vi "Dashboard Main.vi"() -> ()   [LabVIEW 2015]
uses:
  <vilib>/Utility/miscctls.llb/LVRowAndColumnTypeDef.ctl
  <vilib>/event_ctls.llb/eventvkey.ctl
  <vilib>/Rock Robotics/Network Tables/NT Read Boolean.vi
  <vilib>/Rock Robotics/WPI/Dashboard/WPI_DashboardLogging Global.vi
  <vilib>/Rock Robotics/Network Tables/NT Read Numeric Array.vi
  <vilib>/Utility/config.llb/Write Key (String).vi
  <vilib>/Utility/config.llb/Write Key (I32).vi
  <vilib>/Rock Robotics/Network Tables/NT Write Boolean.vi
  <vilib>/Utility/config.llb/NI_LVConfig.lvlib
panel:
  out "Gyro":dbl(knob)=-1.8413610199999755 scale=-180.0..180.0
  in  "Auto Delay (s)":dbl
  in  "Select Auto":string(combo)="Cross" caption="I don't care if I have the routine you want,\nCLICK ME AGAIN"
  out "Binary Image":T1(plugin-control)
  in  "TCP":refnum<k5>
  out "Camera IP":string="0.0.0.0"
  out "Image Message":string="Timeout in Camera Communications"
  in  "Dashboard Tab":T2(tab)
  in  "Cross Back":bool
  in  "Defense":u16(ring) items=["Default", "Low Bar", "Portcullis", "Cheval de Frise", "Ramparts", "Moat", "Drawbridge", "Sally Port", "Rock Wall", "Rough Terrain"]
  in  "Joystick Drive":u16(ring) items=["TANK DRIVE", "LEFT ARCADE", "RIGHT ARCADE"]
  in  "Auto Routine":u16(ring)=1 items=["Do Nothing", "Cross", "Spybot", "Reach", "Test"]
  in  "Shoot?":bool=TRUE
  in  "Defense Position":dbl=1.0 min=0.0 max=5.0 format="%#_1g"
  in  "Camera Settings":T3={"Frame Rate"=15, "Compression"=30, "Size"=1} {"Frame Rate" scale=1.0..30.0; "Size" items=["640x480", "320x240", "160x120"]}
  out "Mode":T4(ring)=enum."Disconnected"
  in  "DB Camera Config":bool
  out "fps":dbl=0.2739425816348893 format="%#.1g"
  out "Mbps":dbl=2.2448263767099263e-06 format="%#.1g"
  out "Mbps LED":bool
  in  "Rec Mode":enum32{"Stop", "Record", "Playback"}(radio)
  out "NT Connection":bool=TRUE
  in  "Vision":u16(ring)=2 items=["Camera Off", "USB Camera SW", "USB Camera HW", "IP Camera"]
  out "Time Left":string="135"
  out "Background":bool=TRUE
  in  "DB/String 9":string
  in  "DB/String 8":string
  in  "DB/String 7":string
  in  "DB/String 6":string
  in  "DB/String 5":string
  in  "DB/String 4":string
  in  "DB/String 3":string
  in  "DB/String 2":string
  in  "DB/String 1":string
  in  "DB/String 0":string
  in  "DB/Slider 0":dbl(slide)=1.0 caption="Intake Roller Speed" min=0.0 max=1.0 scale=0.0..1.0
  in  "DB/Slider 1":dbl(slide) scale=0.0..5.0
  in  "DB/Slider 2":dbl(slide) scale=0.0..5.0
  in  "DB/Slider 3":dbl(slide) scale=0.0..5.0
  out "DB/LED 3":bool
  out "DB/LED 2":bool
  out "DB/LED 1":bool
  out "DB/LED 0":bool
  in  "DB/Button 3":bool
  in  "DB/Button 2":bool
  in  "DB/Button 1":bool
  in  "DB/Button 0":bool caption="New Name"
  in  "Test Slider":dbl(slide) scale=0.0..100.0 scale format="%#_3g"
  in  "On/Off":bool caption="Solenoid"
  in  "Test Name":u16(ring) items=["Select the test to run..."]
  in  "Test Tree":string(tree)
  in  "Motor":cluster{"Value":dbl, "Enable":bool} {"Value" scale=-1.0..1.0 scale format="%#_3g"}
  out "Progress":T5 {"Test Progress" scale=0.0..100.0}
  in  "Rev/Fwd":cluster{"Forward":bool, "Reverse":bool}
  in  "Test Ring":u16(ring) items=["Monochrome", "Color"]
  out "Cmd Status":string
  in  "Execute Command":bool
  in  "Command Params":string[][](table)
  in  "Command Selection":i32(listbox)
  in  "CheckList":i32(listbox)
  out "Tree":string(tree)
  out "Camera Image":T1(plugin-control)
  # "1 Low Bar\n2 Porticullis\n3 Cheval De Frise\n4 Ramparts\n5 Moat\n6 Drawbridge\n7 Sally Port\n8 Rock Wall\n9 Rough Terain"
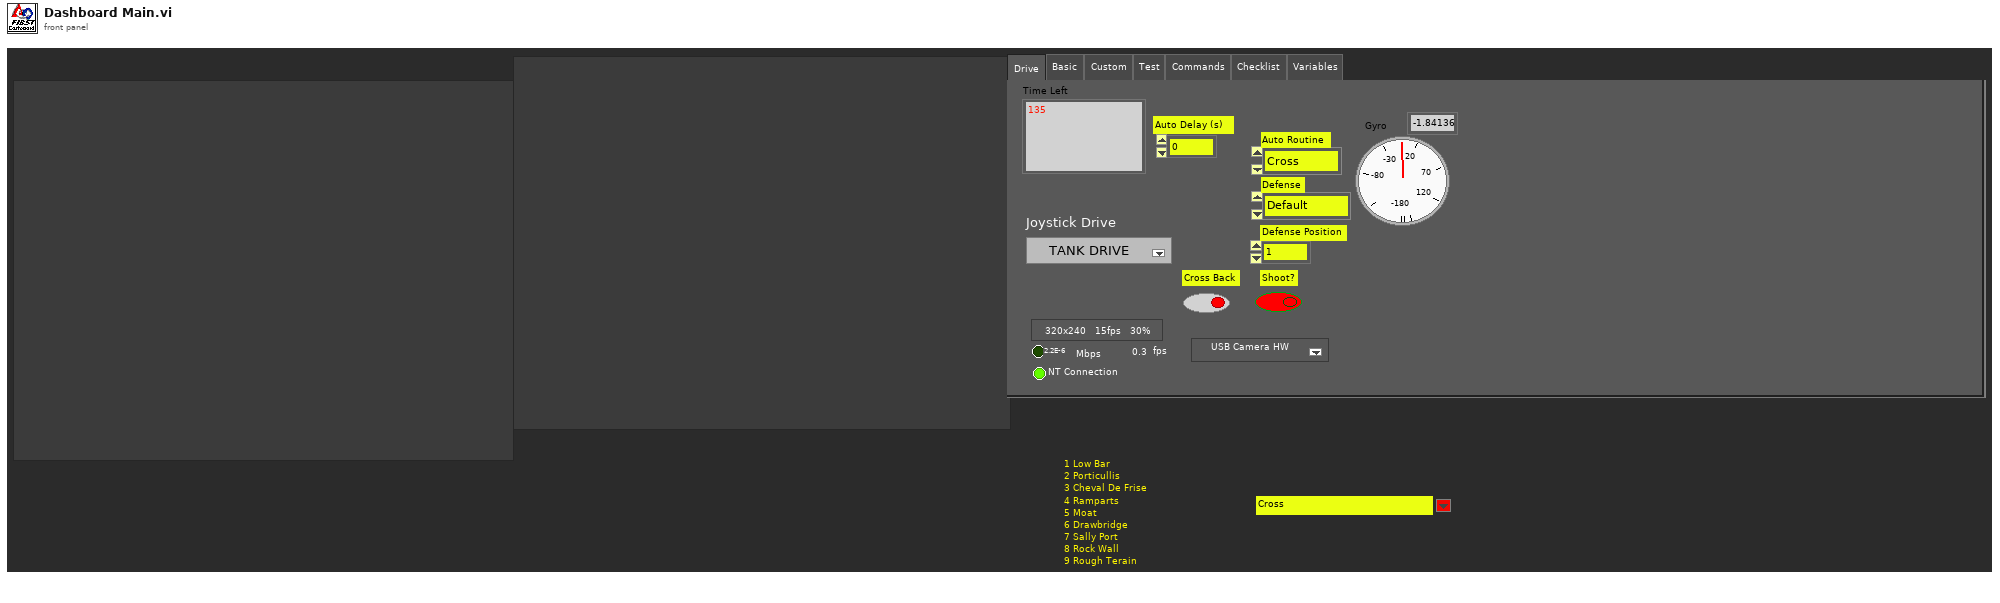
[diagram p1: front panel]
types:
  T1 = typedef "IMAQ Image.ctl" = refnum<image>
  T2 = enum32{"Drive", "Basic", "Custom", "Test", "Commands", "Checklist", "Variables"}
  T3 = cluster{"Frame Rate":i32, "Compression":i32, "Size":u16}
  T4 = enum8{"Tele-Op Disabled", "Tele-Op Enabled", "Auto Disabled", "Auto Enabled", "Test Disabled", "Test Enabled", "Disconnected", "No Code", "E-Stop"}
  T5 = cluster{"Test Progress":u8, "Test Progress Text":string}
  T6 = cluster{"IDs":cluster{"RPC field ID":u16, "Unique ID":u16}, "String":string}
  T7 = enum32{"Drive", "Basic", "Custom", "Test", "Checklist", "Variables"}
  T8 = typedef "Image Type" = u32
  T9 = cluster{"Camera Image":refnum<vi>, "Dashboard Tab":refnum<vi>, "Background":refnum<vi>, "Vision":refnum<vi>, "Rec Mode":refnum<vi>, "Test Slider":refnum<vi>, "On/Off ":refnum<vi>, "Test Ring":refnum<vi>, "Rev/Fwd":refnum<vi>, "Test Name":refnum<vi>, "Motor":refnum<vi>, "Progress":refnum<vi>, "CheckList":refnum<vi>, "Tree":refnum<vi>, "Test Tree":refnum<vi>, "Command Params":refnum<vi>, "Command Selection":refnum<vi>, "Execute Command":refnum<vi>, "Cmd Status":refnum<vi>}
  T10 = cluster{"Bounding box":cluster{"left":dbl, "top":dbl, "right":dbl, "bottom":dbl}, "x":dbl, "y":dbl}
  T11 = cluster{"left":dbl, "top":dbl, "right":dbl, "bottom":dbl}
  T12 = cluster{"x":dbl, "y":dbl, "distance":dbl, "target?":bool}
  T13 = typedef "NI_LVConfig.lvlib/Config Data RefNum.ctl" = refnum<k1>
  T14 = cluster{"Error Strings":string, "Disable Counts":cluster{u16, u16}, "Rail Faults":cluster{u16, u16, u16}, "Robot IP":string, "DB Mode":u8, "Event Info":cluster{"Name":string, "Type":u8, "Number":u16, "Replay":u8}, "Camera Addr":string}
  T15 = cluster{"Storage":cluster{"Disk Free":u64, "RAM Block":u32, "RAM free":u32}, "CPU Utilization":cluster{"CPU % ISR":sgl, "CPU % Time Crit":sgl, "CPU % Timed Str":sgl, "CPU % High":sgl, "CPU % Above":sgl, "CPU % Normal":sgl, "CPU % Low":sgl}, "CAN":cluster{"% Bus Utilization":sgl, "Bus Off Cnt":u32, "TX_FIFO Full Cnt":u32, "Receive Error Cnt":u8, "Transmit Error Cnt":u8}, "HID":cluster{"HID Outputs":u32, "Rumble Low":u16, "Rumble High":u16}[]}
  T16 = cluster{"Status bits":cluster{"Test Mode":bool, "Autonomous":bool, "Enabled":bool, "Code Start":bool, "Brownout":bool, "Reserved 2":bool, "Reserved 3":bool, "E-Stop":bool}, "Code Trace":cluster{"Disabled":bool, "TeleOp":bool, "Auto":bool, "Test":bool}, "Controller Type":enum16{"unknown", "cRIO", "roboRio"}, "Code?":enum16{"unknown", "noCode", "code"}, "Battery V":dbl}
  T17 = cluster{"Control Bits":cluster{"TestMode":bool, "Autonomous":bool, "Enabled":bool, "FMS Present":bool, bool, bool, bool, "E-Stop":bool}, "Team Station ":u8, "Countdown":sgl, "Joystick Values":cluster{"Axes":dbl[], "Buttons":bool[], "POVs":i16[]}[]}
  T18 = cluster{"Axes":dbl[], "Buttons":bool[], "POVs":i16[]}[]
  T19 = cluster{"Axes":dbl[], "Buttons":bool[], "POVs":i16[]}
  T20 = cluster{"Operation":enum16{"Update", "Clear"}, "Color Box":u32}[]
  T21 = typedef "eventvkey.ctl" = enum16{"ASCII", "Enter", "Return", "Shift", "Ctrl", "Alt", "Cmd", "Opt", "Caps", "NumLock", "Clear", "Break", "Up", "Down", "Left", "Right", "Insert", "Delete", "Home", "End", "PageUp", "PageDown", "Escape", "Help", "Pause", "ScrollLock", "F1", "F2", "F3", "F4", "F5", "F6", "F7", "F8", "F9", "F10", "F11", "F12", "F13", "F14", "F15", "F16", "F17", "F18", "F19", "F20", "F21", "F22", "F23", "F24", "Play", "VolumeUp", "VolumeDown", "Mute", "Two Byte Char"}
  T22 = cluster{"Image Size":bool, "Image Type":bool, "Pixel Value":bool, "ROI Information":bool, "Zoom Factor":bool}
  T23 = enum8{"Enabled", "Disabled", "Disabled and Grayed Out"}
  T24 = cluster{"Operation":enum16{"Update", "Clear"}, "Color Box":u32}
  T25 = typedef "LVRowAndColumnTypeDef.ctl" = cluster{"Row":i32, "Column":i32}
  T26 = cluster{"Shift":bool, "Ctrl":bool, "Alt":bool, "Cmd":bool, "Opt":bool}
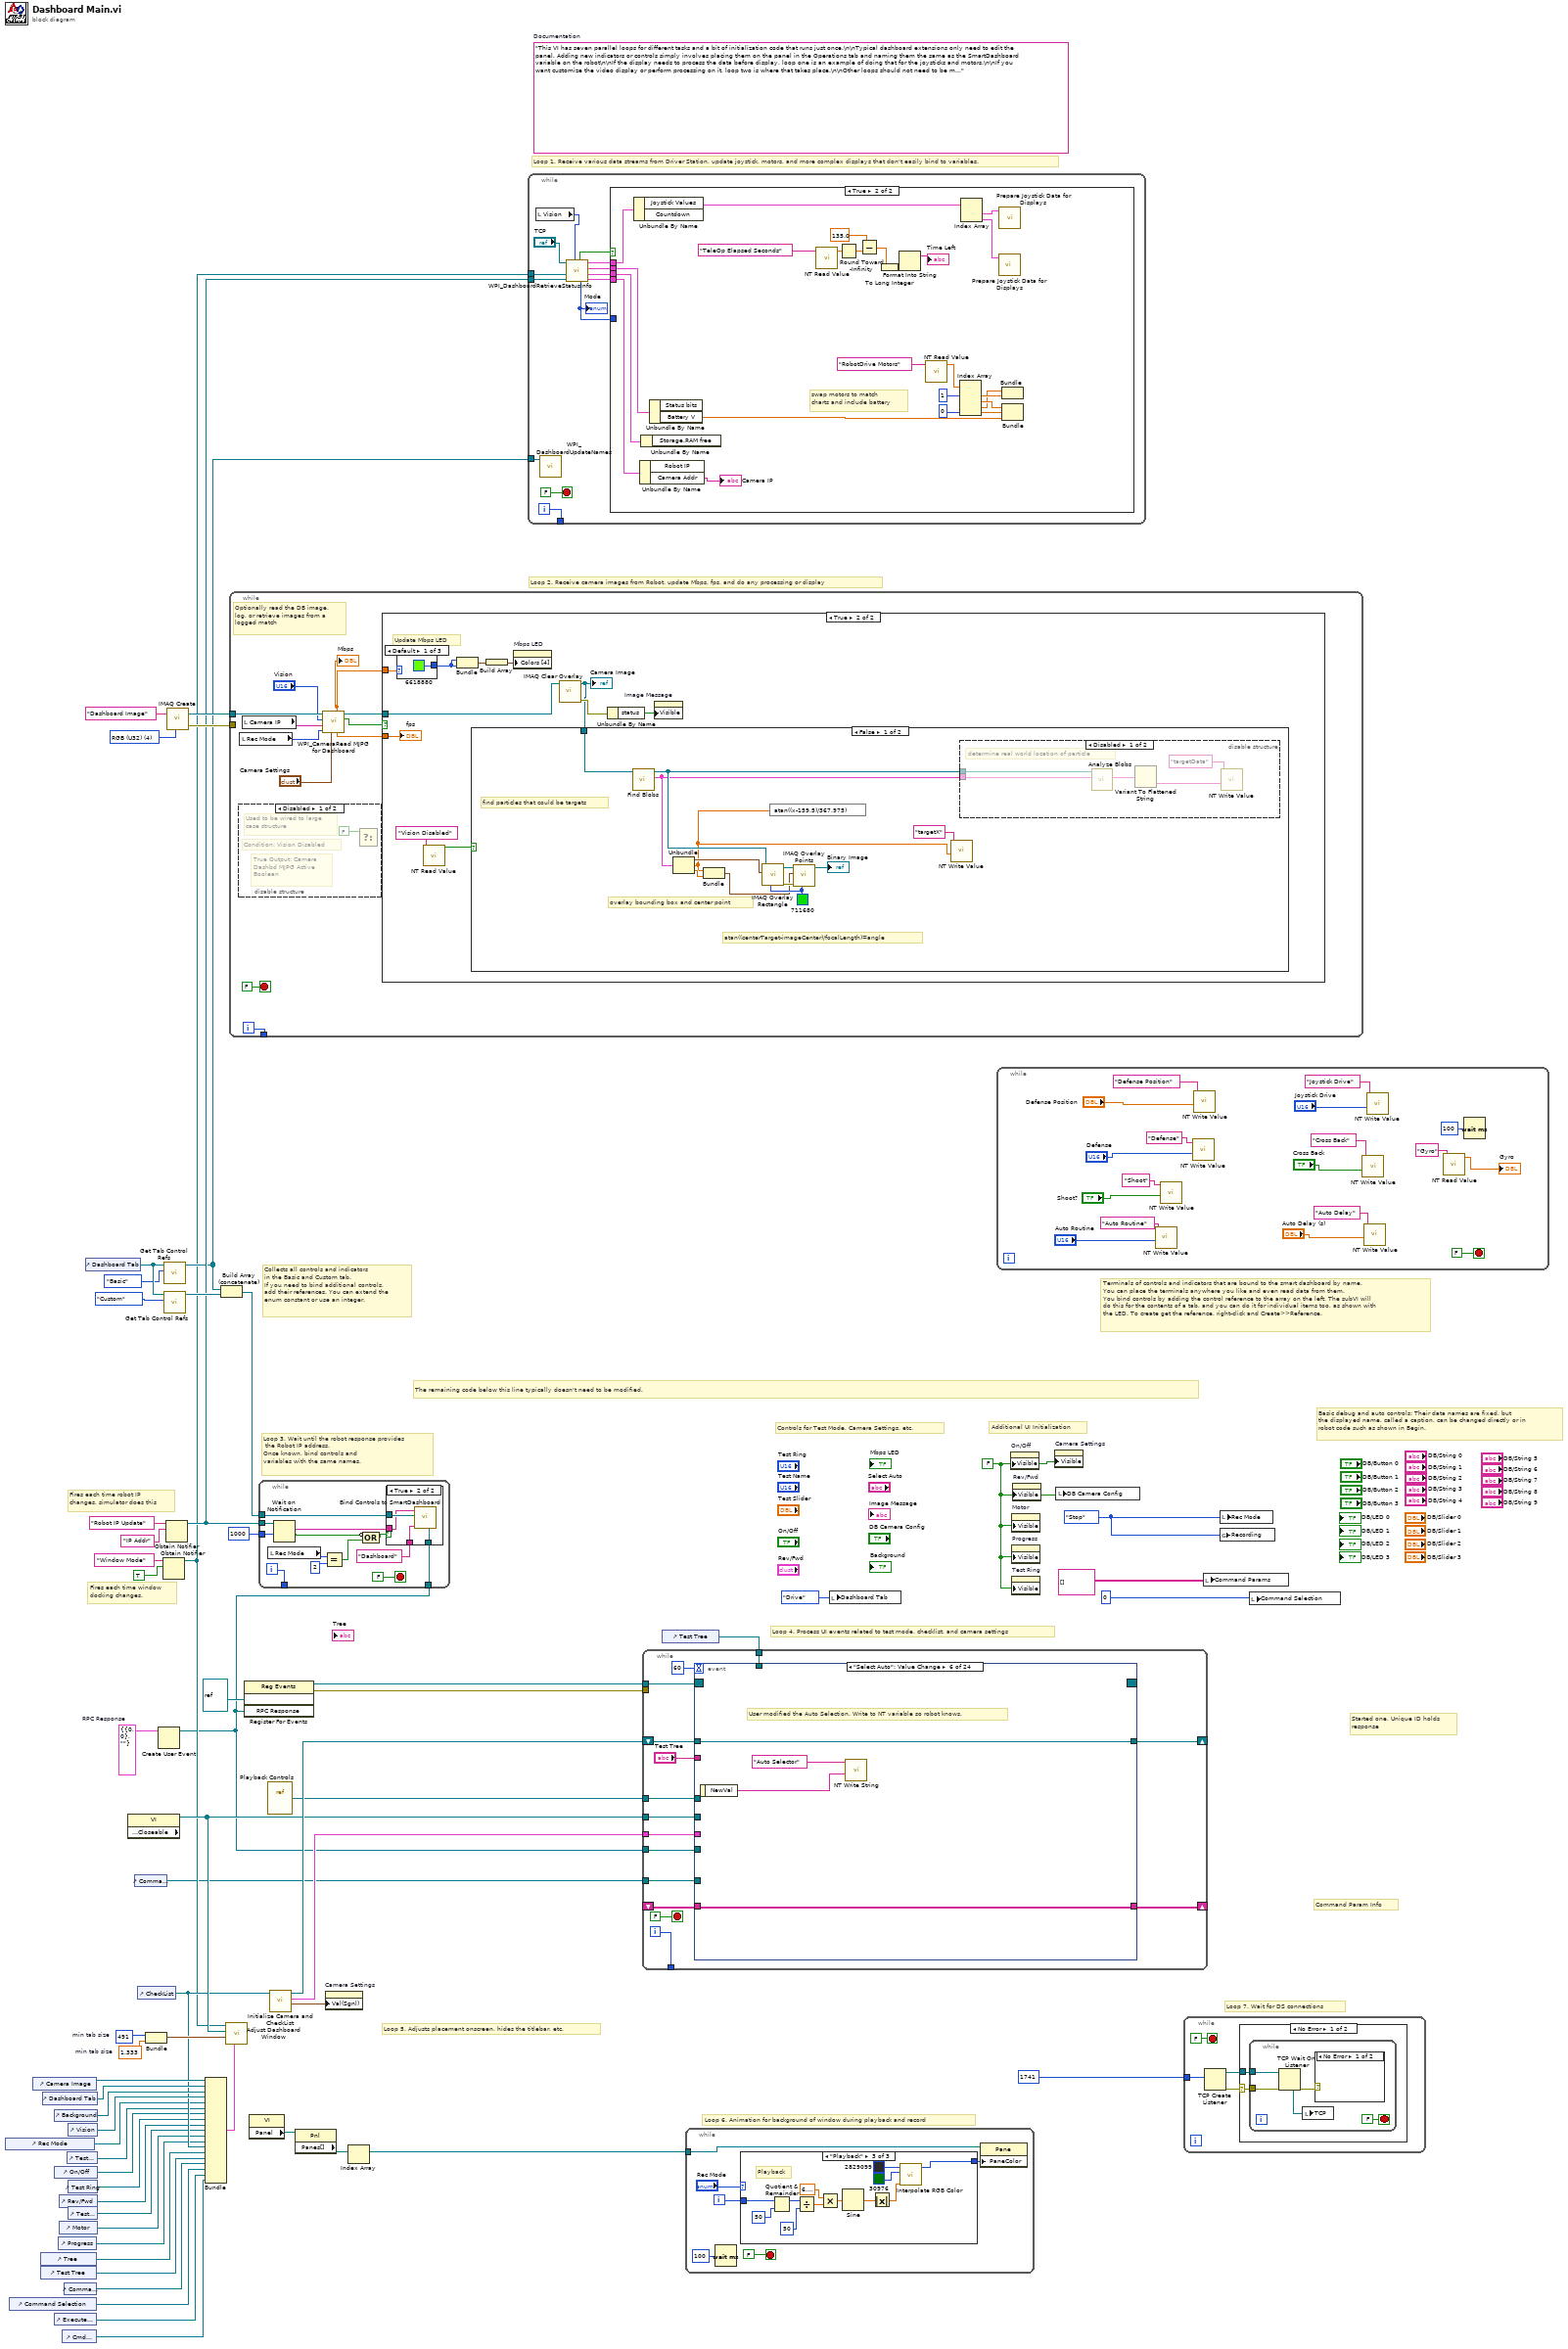
[diagram p0: block diagram]
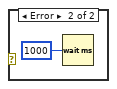
[diagram p2: hidden frame]
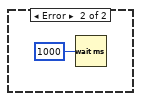
[diagram p3: hidden frame]
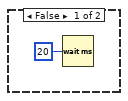
[diagram p4: hidden frame]
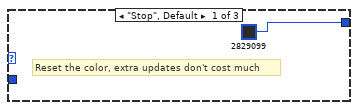
[diagram p5: hidden frame]
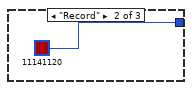
[diagram p6: hidden frame]
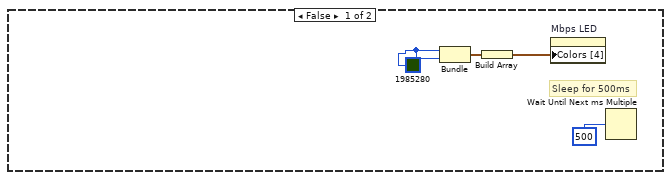
[diagram p9: hidden frame]
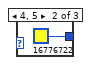
[diagram p12: hidden frame]
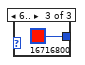
[diagram p13: hidden frame]
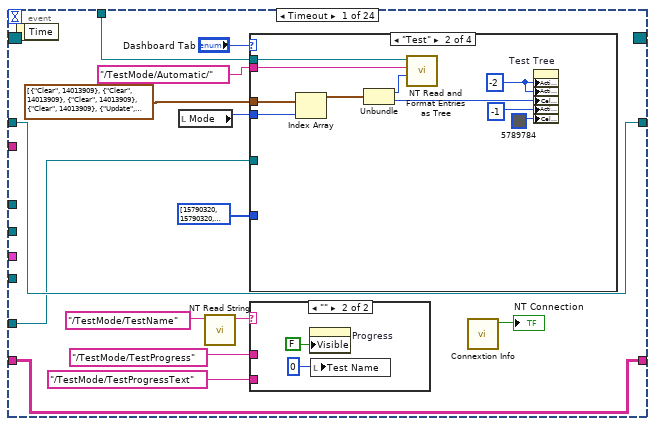
[diagram p14: hidden frame]
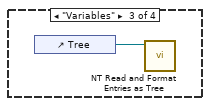
[diagram p16: hidden frame]
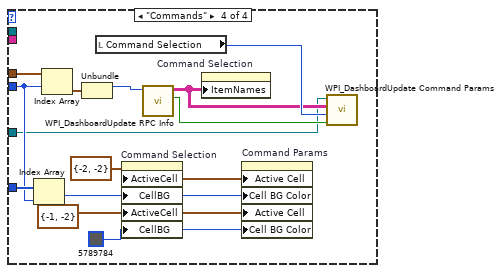
[diagram p17: hidden frame]
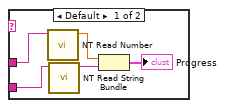
[diagram p18: hidden frame]
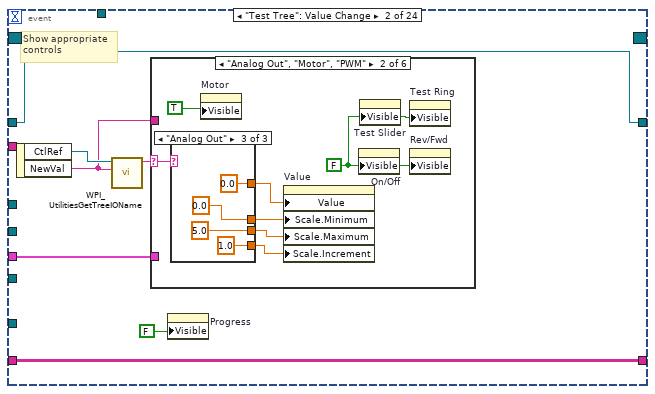
[diagram p19: hidden frame]
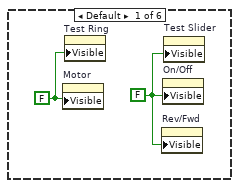
[diagram p20: hidden frame]
diagram:
  w7 = T6 {"IDs"={"RPC field ID"=0, "Unique ID"=0}, "String"=""}  # RPC Response
  w33 = 491  # min tab size
  w32 = 1.333  # min tab size
  w41 = enum32{"Stop", "Record", "Playback"}."Stop" ("Rec Mode")
  w15 = FALSE ("Visible")
  (unwired) "This VI has seven parallel loops for different tasks and a bit of initialization code that runs just once.\n\nTypical dashboard extensions only need to edit the panel. Adding new indicators or controls simply involves placing them on the panel in the Operations tab and naming them the same as the SmartDashboard variable on the robot\n\nIf the display needs to process the data before display, loop one is an example of doing that for the joysticks and motors.\n\nIf you want customize the video display or perform processing on it, loop two is where that takes place.\n\nOther loops should not need to be modified. They are pretty standard, and document the task they perform."  # Documentation
  w61 = T8 4 items=["Grayscale (U8)", "Grayscale (I16)", "Grayscale (SGL)", "Complex (CSG)", "RGB (U32)", "HSL (U32)", "RGB (U64)"] ("Image Type")
  # "Command Param Info"
  # "Started one, Unique ID holds\nresponse"
  # "Loop 7. Wait for DS connections"
  # "Basic debug and auto controls: Their data names are fixed, but\nthe displayed name, called a caption, can be changed directly or in\nrobot code such as shown in Begin."
  # "Controls for Test Mode, Camera Settings, etc."
  # "Additional UI Initialization"
  # "Loop 6. Animation for background of window during playback and record"
  # "Fires each time robot IP\nchanges, simulator does this"
  # "Fires each time window\ndocking changes."
  # "Collects all controls and indicators\nin the Basic and Custom tab.\nIf you need to bind additional controls,\nadd their references. You can extend the\nenum constant or use an integer."
  # "The remaining code below this line typically doesn't need to be modified."
  # "Loop 4. Process UI events related to test mode, checklist, and camera settings"
  # "Terminals of controls and indicators that are bound to the smart dashboard by name.\nYou can place the terminals anywhere you like and even read data from them.\nYou bind controls by adding the control reference to the array on the left. The subVI will\ndo this for the contents of a tab, and you can do it for individual items too, as shown with\nthe LED. To create get the reference, right-click and Create>>Reference."
  # "Loop 3. Wait until the robot response provides\n the Robot IP address.\nOnce known, bind controls and\nvariables with the same names."
  # "Loop 5. Adjusts placement onscreen, hides the titlebar, etc."
  # "Loop 1. Receive various data streams from Driver Station, update joystick, motors, and more complex displays that don't easily bind to variables."
  # "Loop 2. Receive camera images from Robot, update Mbps, fps, and do any processing or display"
  n1 = control-ref of="Rec Mode"() -> (w21:refnum<vi>)
  n2 = control-ref of="Command Selection"() -> (w6:refnum<vi>)
  n3 = control-ref of="Camera Image"() -> (w36:refnum<vi>)
  n4 = control-ref of="Tree"() -> (w25:refnum<vi>)
  n5 = control-ref of="Test Tree"() -> (w24:refnum<vi>)
  n6 = control-ref of="Dashboard Tab"() -> (w35:refnum<vi>)
  n7 = control-ref of="Execute Command"() -> (w8:refnum<vi>)
  n8 = control-ref of="Background"() -> (w30:refnum<vi>)
  n9 = control-ref of="On/Off"() -> (w19:refnum<vi>)
  n10 = control-ref of="Progress"() -> (w16:refnum<vi>)
  n11 = control-ref of="Rev/Fwd"() -> (w17:refnum<vi>)
  n12 = control-ref of="Motor"() -> (w22:refnum<vi>)
  n13 = control-ref of="Cmd Status"() -> (w2:refnum<vi>)
  n14 = control-ref of="Command Params"() -> (w9:refnum<vi>)
  n15 = control-ref of="Test Slider"() -> (w20:refnum<vi>)
  n16 = control-ref of="Vision"() -> (w34:refnum<vi>)
  n17 = control-ref of="Test Ring"() -> (w18:refnum<vi>)
  n18 = control-ref of="Test Name"() -> (w23:refnum<vi>)
  n19 = control-ref of="Dashboard Tab"() -> (w39:refnum<vi>)
  n20 = property class="VI" props=["Front Panel.Closeable"]() -> (reference out=w40:refnum<vi>)  [unwired: 2 in, 2 out]
  n21 = control-ref of="Command Params"() -> (w1:refnum<vi>)
  n22 = control-ref of="CheckList"() -> (w26:refnum<vi>)
  n23 = Bundle("min tab size"=w33, "min tab size"=w32) -> (w31:cluster{"min tab size":i32, "min tab size":dbl})  [unwired: 1 in]
  n24 = Create User Event(user event datatype=w7) -> (user event=w3:refnum<user-event>)  [unwired: 1 in, 1 out]
  n25 = Obtain Notifier(name (unnamed)="Window Mode", notification data type=TRUE) -> (notifier out=w12:refnum<notifier>)  [unwired: 2 in, 2 out]
  n26 = call <vilib>:"Get Tab Control Refs.vi"("Page Index"=T7."Basic" ("Dashboard Tab"), "TabControl in"=w39) -> ("ControlsOnPage"=w13:refnum<vi>[])  [unwired: 9 in]
  n27 = call <vilib>:"Get Tab Control Refs.vi"("Page Index"=T7."Custom" ("Dashboard Tab"), "TabControl in"=w39) -> ("ControlsOnPage"=w38:refnum<vi>[])  [unwired: 9 in]
  n28 = Obtain Notifier(name (unnamed)="Robot IP Update", notification data type="IP Addr" ("name (unnamed)")) -> (notifier out=w14:refnum<notifier>)  [unwired: 2 in, 2 out]
  n29 = call "IMAQ Create"("Image Name"="Dashboard Image", "Image Type"=w61) -> ("New Image"=w59:T1, "error out"=w58:errorcluster)  [unwired: 2 in, 1 out]
  n30 = Bundle("Camera Image"=w36, "Dashboard Tab"=w35, "Background"=w30, "Vision"=w34, "Rec Mode"=w21, "Test Slider"=w20, "On/Off"=w19, "Test Ring"=w18, "Rev/Fwd"=w17, "Test Name"=w23, "Motor"=w22, "Progress"=w16, "CheckList"=w26, "Tree"=w25, "Test Tree"=w24, "Command Params"=w9, "Command Selection"=w6, "Execute Command"=w8, "Cmd Status"=w2) -> (w27:T9)  [unwired: 1 in]
  n31 = Build Array (concatenate)(w13, w38) -> (w37:refnum<vi>[])
  n32 = call "Adjust Dashboard Window.vi"("Sizing Refnums"=w27, "Size Constraints"=w31, "VI"=w40, "WIn Mode"=w12) -> ()  [unwired: 8 in]
  n33 = while {
    tunnel: w59 -> [w70]
    tunnel: w58 -> [_]
    tunnel: [w71] -> _
    i -> [w71]
    stop <- FALSE stop-if-true
    # "Optionally read the DB image,\nlog, or retrieve images from a\nlogged match"
    n34 = disable-structure shown="Disabled" {
      frame Disabled {
        # "Used to be wired to large\ncase structure"
        # "True Output: Camera\nDashbd MJPG Active\nBoolean"
        # "Condition: Vision Disabled"
        n35 = Select(t=FALSE) -> ()  [unwired: 2 in, 1 out]
      }
      frame Enabled {
      }
    }
    n36 = local read "Rec Mode"() -> (w67:enum32{"Stop", "Record", "Playback"})
    n37 = local read "Camera IP"() -> (w64:string)
    n38 = call <vilib>:"WPI_CameraRead MJPG for Dashboard.vi"("Camera Settings"="Camera Settings", "Rec Mode"=w67, "Camera IP"=w64, "Camera Mode"="Vision", "Refnum in"=w70) -> ("Active"=w62:bool, "Refnum out"=w69:T1, "FPS"=w68:dbl, "Bandwidth (Mbps)"=w66:dbl)  [unwired: 3 in]
    "Mbps" <- w66
    n39 = case shown="True" w62 {
      tunnel: w69 -> [_ w83]
      tunnel: w66 -> [_ w82]
      tunnel: w68 -> [_ w79]
      frame False {
        w74 = u32 1985280 ("Color Box")
        # "Sleep for 500ms"
        n40 = Bundle("Color Box"=w74, "Color Box"=w74) -> (w76:cluster{"Color Box":u32, "Color Box":u32})  [unwired: 1 out]
        n41 = Build Array(w76) -> (w75:cluster{"Color Box":u32, "Color Box":u32}[])
        n42 = property on="Mbps LED" class="Bool (strict)"("Colors [4]"=w75) -> ()  [unwired: 2 in, 2 out]
        n43 = Wait Until Next ms Multiple(millisecond multiple=u32 500) -> ()  [unwired: 1 out]
      }
      frame True {
        # "Update Mbps LED"
        n44 = case shown="Default" w82 {
          tunnel: [u32 6618880 ("Color Box") u32 16776722 ("Color Box") u32 16716800 ("Color Box")] -> w84
          frame Default {
          }
          frame 4, 5 {
          }
          frame 6.. {
          }
        }
        n45 = call-poly <vilib>:"NT Read Value.vi"("Name"="Vision Disabled") -> ("Boolean"=w80:bool)  [unwired: 9 in, 1 out]
        n46 = Bundle("Color Box"=w84, "Color Box"=w84) -> (w86:cluster{"Color Box":u32, "Color Box":u32})  [unwired: 1 out]
        n47 = Build Array(w86) -> (w85:cluster{"Color Box":u32, "Color Box":u32}[])
        n48 = property on="Mbps LED" class="Bool (strict)"("Colors [4]"=w85) -> ()  [unwired: 2 in, 2 out]
        n49 = call "IMAQ Clear Overlay"("Image"=w83) -> ("error out"=w87:errorcluster, "Image Out"=w78:T1)  [unwired: 2 in, 7 out]
        "Camera Image" <- w78
        n50 = case shown="False" w80 {
          tunnel: w78 -> [w100 _]
          frame False {
            w97 = u32 711680 ("Color")
            # "atan((centerTarget-imageCenter)/focalLength)=angle"
            # "find particles that could be targets"
            # "overlay bounding box and center point"
            n51 = call "Find Blobs.vi"("Image In"=w100) -> ("Blob Data"=w94:T10, "Image Out"=w95:T1)  [unwired: 9 in]
            n52 = Unbundle(w94) -> ("Bounding box"=w93:T11, "x"=w89:dbl, "y"=w92:dbl)
            n53 = Bundle("x"=w89, "y"=w92) -> (w91:cluster{"x":dbl, "y":dbl})  [unwired: 1 in]
            n54 = call "IMAQ Overlay Rectangle"("Color"=w97, "Rectangle"=w93, "Image"=w95) -> ("error out"=w99:errorcluster, "Image Out"=w98:T1)  [unwired: 7 in]
            n55 = expression code="atan((x-159.5)/367.975)"(w89) -> ()  [unwired: 1 out]
            n56 = call "IMAQ Overlay Points"("Color"=w97, "error in (no error)"=w99, "Point"=w91, "Image"=w98) -> ("Image Out"=→"Binary Image":T1)  [unwired: 6 in, 1 out]
            n57 = call-poly <vilib>:"NT Write Value.vi"("Numeric"=w89, "Name"="targetX") -> ()  [unwired: 9 in, 1 out]
            n58 = disable-structure shown="Disabled" {
              disable-tunnel: w95 -> [w104 _]
              disable-tunnel: w94 -> [w103 _]
              frame Disabled {
                # "determine real world location of particle"
                n59 = call "Analyze Blobs.vi"("Image In"=w104, "Blob Data"=w103) -> ("Target Data"=w102:T12)  [unwired: 7 in, 1 out]
                n60 = Variant To Flattened String(Variant=w102) -> (data string=w101:string)  [unwired: 1 out]
                n61 = call-poly <vilib>:"NT Write Value.vi"("String"=w101, "Name"="targetData") -> ()  [unwired: 9 in, 1 out]
              }
              frame Enabled {
              }
            }
          }
          frame True {
          }
        }
        n62 = Unbundle By Name(w87) -> ("status"=w88:bool)
        n63 = property on="Image Message" class="Str"("Visible"=w88) -> ()  [unwired: 2 in, 2 out]
        "fps" <- w79
      }
    }
  }
  n64 = register-events(refnum<vi> refnum, w3) -> (reference out=w45:refnum<event-registration>, error out=w44:errorcluster)  [unwired: 2 in]
  n65 = property class="VI"() -> ("Panel"=w48:refnum<vi>)  [unwired: 2 in, 2 out]
  n66 = while {
    tunnel: w37 -> [w121]
    tunnel: w14 -> [w119]
    tunnel: [w117] -> _
    tunnel: u32 1000 ("milliseconds to wait") -> [w116]
    tunnel: w3 -> [w109]
    i -> [w117]
    stop <- FALSE stop-if-true
    n67 = local read "Rec Mode"() -> (w112:enum32{"Stop", "Record", "Playback"})
    n68 = Wait on Notification(notifier=w119, timeout in ms (-1)=w116) -> (notification=w118:string, timed out?=w114:bool)  [unwired: 2 in, 2 out]
    n69 = Equal?(x=w112, y=u16 2 ("Rec Mode")) -> (x = y?=w113:bool)
    n70 = Compound Arithmetic op=OR(invert w114, w113) -> (w115:bool)
    n71 = case shown="True" w115 {
      tunnel: w121 -> [_ w125]
      tunnel: w118 -> [_ w124]
      tunnel: "Dashboard" -> [_ w123]
      tunnel: w109 -> [_ w122]
      frame False {
      }
      frame True {
        n72 = call <vilib>:"Bind Controls to SmartDashboard.vi"("RPC ref"=w122, "Client Name"=w123, "Bound Control Refs"=w125, "Server IP Address"=w124) -> ()  [unwired: 8 in]
      }
    }
  }
  n73 = vi-ref "Playback Controls.vi"() -> (w46:refnum<vi>)
  n74 = call "Initialize Camera and CheckList.vi"("ListBox in"=w26) -> ("Cluster"=w52:cluster{"value":i32, "value":i32, "index":i32}, "Array"=w53:cluster{string[]}[], "File Refnum"=w51:T13)  [unwired: 8 in]
  n75 = property class="Pnl"(reference=w48) -> ("Panes[]"=w49:refnum<vi>[])  [unwired: 1 in, 2 out]
  n76 = property on="Camera Settings" class="Clust (strict)"("Val(Sgnl)"=w52) -> ()  [unwired: 2 in, 2 out]
  n77 = Index Array(array=w49) -> (element=w47:refnum<vi>)  [unwired: 1 in]
  n78 = while {
    tunnel: [w137] -> _
    tunnel: w14 -> [w131]
    tunnel: w13 -> [w130]
    tunnel: w12 -> [w126]
    i -> [w137]
    stop <- FALSE stop-if-true
    n79 = local read "Vision"() -> (w128:u16)
    n80 = call <vilib>:"WPI_DashboardUpdateNames.vi"("Controls on Tab"=w130) -> ()  [unwired: 11 in]
    n81 = call <vilib>:"WPI_DashboardRetrieveStatusInfo.vi"("Vision"=w128, "Binding Refnum"=w131, "Window Mode Notifier"=w126, "TCP Cnx"="TCP") -> ("Power and Errors"=w132:T14, "Robot Metrics"=w135:T15, "Status Info"=w136:T16, "Control Info"=w133:T17, "Robot Mode"=w129:T4, "Process?"=w134:bool)  [unwired: 2 in]
    "Mode" <- w129
    n82 = case shown="True" w134 {
      tunnel: w136 -> [_ w163]
      tunnel: w135 -> [_ w162]
      tunnel: w133 -> [_ w161]
      tunnel: w132 -> [_ w160]
      tunnel: w129 -> [_ _]
      frame False {
        n83 = Wait (ms)(milliseconds to wait=u32 20) -> ()  [unwired: 1 out]
      }
      frame True {
        # "swap motors to match\ncharts and include battery"
        n84 = Unbundle By Name(w161) -> ("Joystick Values"=w152:T18)  [unwired: 1 out]
        n85 = Unbundle By Name(w160) -> ("Camera Addr"=→"Camera IP":string)  [unwired: 1 out]
        n86 = Unbundle By Name(w162) -> ()  [unwired: 1 out]
        n87 = Unbundle By Name(w163) -> ("Battery V"=w153:dbl)  [unwired: 1 out]
        n88 = call-poly <vilib>:"NT Read Value.vi"("Name"="TeleOp Elapsed Seconds") -> ("Numeric"=w144:dbl)  [unwired: 9 in, 1 out]
        n89 = Round Toward -Infinity(1:w144) -> (0:w143:dbl)
        n90 = Subtract(x=135.0, y=w143) -> (x-y=w140:dbl)
        n91 = To Long Integer(number=w140) -> (32bit integer=w141:i32)
        n92 = Format Into String(w141) -> (resulting string=→"Time Left":string)  [unwired: 3 in, 1 out]
        n93 = call-poly <vilib>:"NT Read Value.vi"("Name"="RobotDrive Motors") -> ("Numeric Array"=w147:dbl[])  [unwired: 9 in, 1 out]
        n94 = Index Array(array=w147, index #1=1, index #4=0) -> (element #1=w155:dbl, element #2=w156:dbl, element #3=w154:dbl, element #4=w159:dbl)  [unwired: 2 in]
        n95 = Index Array(array=w152) -> (element #1=w151:T19, element #2=w149:T19)  [unwired: 2 in]
        n96 = call "Prepare Joystick Data for Displays.vi"("Joystick Values"=w149) -> ()  [unwired: 8 in, 3 out]
        n97 = call "Prepare Joystick Data for Displays.vi"("Joystick Values"=w151) -> ()  [unwired: 8 in, 3 out]
        n98 = Bundle("Numeric"=w154, "Numeric"=w155) -> ()  [unwired: 1 in, 1 out]
        n99 = Bundle("Numeric"=w156, "Numeric"=w159, "Battery V"=w153) -> ()  [unwired: 1 in, 1 out]
      }
    }
  }
  n100 = control-ref of="Test Tree"() -> (w50:refnum<vi>)
  n101 = while {
    tunnel: w53 -> [w175]
    shift-right: [w174] -> _
    shift-left: w51 -> [w173]
    tunnel: [w172] -> _
    tunnel: w50 -> [w171]
    tunnel: w46 -> [w170]
    tunnel: w45 -> [w169]
    tunnel: w44 -> [_]
    tunnel: w40 -> [w168]
    tunnel: w3 -> [w167]
    tunnel: w1 -> [w166]
    shift-right: [w165] -> _
    shift-left: _ -> [w164]
    i -> [w172]
    stop <- FALSE stop-if-true
    n102 = event shown="[5] \"Select Auto\": Value Change" {
      selector: w169 -> [_ _ _ _ _ _ _ _ _ _ _ _ _ _ _ _ _ _ _ _ _ _ _ _]
      dyn-events: [_ _ _ _ _ _ _ _ _ _ _ _ _ _ _ _ _ _ w484 _ _ _ _ _] -> _
      timeout: u32 60 ("milliseconds to wait") -> [_ _ _ _ _ _ _ _ _ _ _ _ _ _ _ _ _ _ _ _ _ _ _ _]
      tunnel: w171 -> [w188 _ _ _ _ _ _ _ _ _ _ _ _ _ _ _ _ _ _ _ _ _ _ _]
      tunnel: "Test Tree" -> [_ _ _ _ _ _ _ _ _ _ _ _ _ w447 w456 w459 w464 w473 _ _ _ _ _ _]
      tunnel: w175 -> [_ w226 _ _ _ _ _ _ _ _ _ w409 w440 _ _ _ _ _ _ _ _ _ _ _]
      tunnel: [w185 w225 w329 w335 w345 w349 w355 w367 w375 w381 w394 w408 w433 w446 w454 w458 w463 w472 w486 w502 w504 w512 w523 w528] -> w174
      tunnel: w173 -> [w185 w225 w329 w335 w345 w349 w355 w367 w375 w381 w394 w407 w433 w446 w454 w458 w463 w472 w486 w502 w504 w512 w523 w528]
      tunnel: w170 -> [_ _ _ _ _ _ _ _ _ _ _ _ _ _ _ _ _ _ w487 _ w507 _ _ _]
      tunnel: w168 -> [_ _ _ _ _ _ _ _ _ _ _ _ _ _ _ _ _ _ w482 _ _ _ _ _]
      tunnel: w167 -> [_ _ _ _ _ _ _ _ _ _ _ _ _ _ _ _ _ _ w478 _ _ _ _ _]
      tunnel: w166 -> [w180 _ _ _ _ _ w353 _ _ _ _ _ _ _ _ _ _ _ _ _ _ _ _ _]
      tunnel: [w179 w224 w328 w334 w344 w350 w351 w361 w372 w380 w393 w406 w432 w445 w453 w457 w462 w471 w477 w500 w503 w508 w516 w529] -> w165
      tunnel: w164 -> [w179 w224 w328 w334 w344 w350 w351 _ _ w380 w393 w406 w432 w445 w453 w457 w462 w471 w477 w500 w503 w508 w516 w529]
      event Timeout {
        n103 = event-data() -> ()  [unwired: 1 in, 1 out]
        n104 = local read "Mode"() -> (w182:T4)
        n105 = call <vilib>:"NT Read String.vi"("Name"="/TestMode/TestName") -> ("String"=w191:string)  [unwired: 9 in, 1 out]
        n106 = case shown="\"Test\"" "Dashboard Tab" {
          tunnel: w188 -> [_ w202 _ _]
          tunnel: "/TestMode/Automatic/" ("Name Pattern") -> [_ w201 _ _]
          tunnel: T20 [{"Operation"=enum."Clear", "Color Box"=14013909}, {"Operation"=enum."Clear", "Color Box"=14013909}, {"Operation"=enum."Clear", "Color Box"=14013909}, {"Operation"=enum."Clear", "Color Box"=14013909}, {"Operation"=enum."Update", "Color Box"=14013909}, {"Operation"=enum."Update", "Color Box"=16777215}, {"Operation"=enum."Clear", "Color Box"=14013909}, {"Operation"=enum."Clear", "Color Box"=14013909}, {"Operation"=enum."Clear", "Color Box"=14013909}] -> [_ w194 _ w211]
          tunnel: w182 -> [_ w193 _ w210]
          tunnel: u32[] [15790320, 15790320, 15790320, 15790320, 16777215, 16777215, 15790320, 15790320, 15790320] -> [_ _ _ w216]
          tunnel: w180 -> [_ _ _ w204]
          frame "Custom", Default {
          }
          frame "Test" {
            w200 = -2 ("Active Item:Row Number")
            n107 = Index Array(array=w194, index=w193) -> (element=w195:T24)
            n108 = Unbundle(w195) -> ("Operation"=w196:enum16{"Update", "Clear"}, "Color Box"=w197:u32)
            n109 = call <vilib>:"NT Read and Format Entries as Tree.vi"("Operation"=w196, "Name Pattern"=w201, "Tree Refnum"=w202) -> ()  [unwired: 7 in, 2 out]
            n110 = property on="Test Tree" class="Tree (strict)"("Active Item Row Number"=w200, "ActiveColNum"=w200, "CellBG"=w197, "Active Item Row Number"=-1 ("Active Item:Row Number"), "CellBG"=u32 5789784 ("Color Box")) -> ()  [unwired: 2 in, 2 out]
          }
          frame "Variables" {
            n111 = control-ref of="Tree"() -> (w203:refnum<vi>)
            n112 = call <vilib>:"NT Read and Format Entries as Tree.vi"("Tree Refnum"=w203) -> ()  [unwired: 9 in, 2 out]
          }
          frame "Commands" {
            w212 = u32 5789784 ("Color Box")
            w213 = T25 {"Row"=-1, "Column"=-2} ("Active Cell:Active Cell")
            w215 = T25 {"Row"=-2, "Column"=-2} ("Active Cell:Active Cell")
            n113 = Index Array(array=w216, index=w210) -> (element=w214:u32)
            n114 = Index Array(array=w211, index=w210) -> (element=w209:T24)
            n115 = Unbundle(w209) -> ("Operation"=w208:enum16{"Update", "Clear"})  [unwired: 1 out]
            n116 = local read "Command Selection"() -> (w207:i32)
            n117 = property on="Command Selection" class="MCListbox (strict)"("ActiveCell"=w215, "CellBG"=w214, "ActiveCell"=w213, "CellBG"=w212) -> ()  [unwired: 2 in, 2 out]
            n118 = call <vilib>:"WPI_DashboardUpdate RPC Info.vi"("Operation"=w208) -> ("update"=w206:bool, "commands"=w205:string[][])  [unwired: 9 in]
            n119 = property on="Command Selection" class="MCListbox (strict)"("ItemNames"=w205) -> ()  [unwired: 2 in, 2 out]
            n120 = property on="Command Params" class="Tbl (strict)"("Active Cell"=w215, "Cell BG Color"=w214, "Active Cell"=w213, "Cell BG Color"=w212) -> ()  [unwired: 2 in, 2 out]
            n121 = call <vilib>:"WPI_DashboardUpdate Command Params.vi"("Update"=w206, "NewVal"=w207, "Commands"=w205, "Param Tbl"=w204) -> ()  [unwired: 7 in, 1 out]
          }
        }
        n122 = case shown="\"\"" w191 {
          tunnel: "/TestMode/TestProgress" ("Name") -> [w218 _]
          tunnel: "/TestMode/TestProgressText" ("Name") -> [w217 _]
          frame Default {
            n123 = call <vilib>:"NT Read Number.vi"("Name"=w218) -> ("Numeric"=w219:dbl)  [unwired: 9 in, 1 out]
            n124 = call <vilib>:"NT Read String.vi"("Name"=w217) -> ("String"=w220:string)  [unwired: 9 in, 1 out]
            n125 = Bundle("Numeric"=w219, "String"=w220) -> (→"Progress":cluster{"Numeric":dbl, "String":string})  [unwired: 1 in]
          }
          frame "" {
            n126 = property on="Progress" class="Clust (strict)"("Visible"=FALSE) -> ()  [unwired: 2 in, 2 out]
            n127 = local write "Test Name"(u16 0) -> ()
          }
        }
        n128 = call <vilib>:"Connextion Info.vi"() -> ("Connected"=→"NT Connection":bool)  [unwired: 10 in, 1 out]
      }
      event "Test Tree": Value Change {
        # "Show appropriate\ncontrols"
        n129 = event-data() -> ("CtlRef"=w229:refnum<vi>, "NewVal"=w227:string)  [unwired: 1 in]
        n130 = call <vilib>:"WPI_UtilitiesGetTreeIOName.vi"("NewVal"=w227, "TreeControl in"=w229) -> ("I/O Name"=w230:string)  [unwired: 9 in]
        n131 = case shown="\"Analog Out\", \"Motor\", \"PWM\"" w230 {
          selector: w230 -> [_ w237 _ w259 w268 _]
          tunnel: w227 -> [_ _ w256 w258 _ w275]
          tunnel: w226 -> [_ _ _ _ _ w274]
          frame Default {
            w232 = FALSE ("Visible")
            w231 = FALSE ("Visible")
            n132 = property on="Motor" class="Clust (strict)"("Visible"=w231) -> ()  [unwired: 2 in, 2 out]
            n133 = property on="Test Ring" class="Ring (strict)"("Visible"=w231) -> ()  [unwired: 2 in, 2 out]
            n134 = property on="Rev/Fwd" class="Clust (strict)"("Visible"=w232) -> ()  [unwired: 2 in, 2 out]
            n135 = property on="On/Off" class="Bool (strict)"("Visible"=w232) -> ()  [unwired: 2 in, 2 out]
            n136 = property on="Test Slider" class="Slide (strict)"("Visible"=w232) -> ()  [unwired: 2 in, 2 out]
          }
          frame "Analog Out", "Motor", "PWM" {
            w238 = FALSE ("Visible")
            n137 = case shown="\"Analog Out\"" w237 {
              tunnel: [1.0 ("Value") -1.0 ("Value") 0.0 ("Value")] -> w236
              tunnel: [255.0 ("Value") 1.0 ("Value") 5.0 ("Value")] -> w235
              tunnel: [128.0 ("Value") 0.0 ("Value") 0.0 ("Value")] -> w234
              tunnel: [64.0 ("Value") 0.5 ("Value") 1.0 ("Value")] -> w233
              frame "PWM" {
              }
              frame "Motor", Default {
              }
              frame "Analog Out" {
              }
            }
            n138 = property on="Motor" class="Clust (strict)"("Visible"=TRUE) -> ()  [unwired: 2 in, 2 out]
            n139 = property on="Value" class="Slide (strict)"("Value"=w234, "Scale.Minimum"=w236, "Scale.Maximum"=w235, "Scale.Increment"=w233) -> ()  [unwired: 2 in, 2 out]
            n140 = property on="On/Off" class="Bool (strict)"("Visible"=w238) -> ()  [unwired: 2 in, 2 out]
            n141 = property on="Test Slider" class="Slide (strict)"("Visible"=w238) -> ()  [unwired: 2 in, 2 out]
            n142 = property on="Test Ring" class="Ring (strict)"("Visible"=w238) -> ()  [unwired: 2 in, 2 out]
            n143 = property on="Rev/Fwd" class="Clust (strict)"("Visible"=w238) -> ()  [unwired: 2 in, 2 out]
          }
          frame "Servo" {
            w254 = FALSE ("Visible")
            n144 = call <vilib>:"NT Read Number.vi"("Name"=w256) -> ("Numeric"=w255:dbl)  [unwired: 9 in, 1 out]
            n145 = property on="Test Slider" class="Slide (strict)"("Visible"=TRUE, "Scale.Maximum"=170.0 ("Scale.Range:Maximum")) -> ()  [unwired: 2 in, 2 out]
            n146 = local write "Test Slider"(w255) -> ()
            n147 = property on="Motor" class="Clust (strict)"("Visible"=w254) -> ()  [unwired: 2 in, 2 out]
            n148 = property on="Rev/Fwd" class="Clust (strict)"("Visible"=w254) -> ()  [unwired: 2 in, 2 out]
            n149 = property on="On/Off" class="Bool (strict)"("Visible"=w254) -> ()  [unwired: 2 in, 2 out]
            n150 = property on="Test Ring" class="Ring (strict)"("Visible"=w254) -> ()  [unwired: 2 in, 2 out]
          }
          frame "Relay", "Solenoid" {
            w257 = FALSE ("Visible")
            n151 = property on="Motor" class="Clust (strict)"("Visible"=w257) -> ()  [unwired: 2 in, 2 out]
            n152 = property on="Test Slider" class="Slide (strict)"("Visible"=w257) -> ()  [unwired: 2 in, 2 out]
            n153 = Search and Replace String(input string=w258, search string="/Value  **", replace string="/Direction") -> (result string=w264:string)  [unwired: 5 in, 3 out]
            n154 = property on="Test Ring" class="Ring (strict)"("Visible"=w257) -> ()  [unwired: 2 in, 2 out]
            n155 = call <vilib>:"NT Read String.vi"("Name"=w264) -> ("String"=w262:string)  [unwired: 9 in, 1 out]
            n156 = Equal?(x="Both directions", y=w262) -> (x = y?=w260:bool)
            n157 = Not(x=w260) -> (.not. x?=w261:bool)
            n158 = property on="Rev/Fwd" class="Clust (strict)"("Visible"=w260) -> ()  [unwired: 2 in, 2 out]
            n159 = property on="On/Off" class="Bool (strict)"("Visible"=w261, "Caption.Text"=w259) -> ()  [unwired: 2 in, 2 out]
          }
          frame "Compressor", "Digital Out" {
            w267 = FALSE ("Visible")
            # "Get direction and finish"
            n160 = property on="Motor" class="Clust (strict)"("Visible"=w267) -> ()  [unwired: 2 in, 2 out]
            n161 = property on="Test Slider" class="Slide (strict)"("Visible"=w267) -> ()  [unwired: 2 in, 2 out]
            n162 = property on="Test Ring" class="Ring (strict)"("Visible"=w267) -> ()  [unwired: 2 in, 2 out]
            n163 = property on="On/Off" class="Bool (strict)"("Visible"=TRUE, "Caption.Text"=w268) -> ()  [unwired: 2 in, 2 out]
            n164 = property on="Rev/Fwd" class="Clust (strict)"("Visible"=FALSE) -> ()  [unwired: 2 in, 2 out]
          }
          frame "Camera" {
            n165 = call <vilib>:"Get Last Path Segment.vi"("String in"=w275) -> ("String out"=w276:string)  [unwired: 10 in]
            n166 = property on="On/Off" class="Bool (strict)"("Visible"=FALSE) -> ()  [unwired: 2 in, 2 out]
            n167 = property on="Motor" class="Clust (strict)"("Visible"=FALSE) -> ()  [unwired: 2 in, 2 out]
            n168 = property on="Rev/Fwd" class="Clust (strict)"("Visible"=FALSE) -> ()  [unwired: 2 in, 2 out]
            n169 = case shown="\"White Balance  **\"" w276 {
              tunnel: w275 -> [w282 w291 w300 w309 w318 _ w324]
              tunnel: w274 -> [w280 w288 w297 w306 w315 _ _]
              frame "Size  **" {
                n170 = Index Array(array=w280) -> (element=w279:cluster{string[]})  [unwired: 1 in]
                n171 = call <vilib>:"NT Read String.vi"("Name"=w282) -> ("String"=w281:string)  [unwired: 9 in, 1 out]
                n172 = Unbundle(w279) -> (w277:string[])
                n173 = Match First String(2:w277, 3:w281) -> (0:w278:i32)  [unwired: 1 out]
                n174 = property on="Test Ring" class="Ring (strict)"("Value"=w278, "Strings []"=w277) -> ()  [unwired: 2 in, 2 out]
                n175 = property on="Test Ring" class="Ring (strict)"("Visible"=TRUE) -> ()  [unwired: 2 in, 2 out]
                n176 = property on="Test Slider" class="Slide (strict)"("Visible"=FALSE) -> ()  [unwired: 2 in, 2 out]
              }
              frame "White Balance  **" {
                n177 = Index Array(array=w288, index=1) -> (element=w289:cluster{string[]})
                n178 = call <vilib>:"NT Read String.vi"("Name"=w291) -> ("String"=w290:string)  [unwired: 9 in, 1 out]
                n179 = Unbundle(w289) -> (w286:string[])
                n180 = Match First String(2:w286, 3:w290) -> (0:w285:i32)  [unwired: 1 out]
                n181 = property on="Test Ring" class="Ring (strict)"("Value"=w285, "Strings []"=w286) -> ()  [unwired: 2 in, 2 out]
                n182 = property on="Test Ring" class="Ring (strict)"("Visible"=TRUE) -> ()  [unwired: 2 in, 2 out]
                n183 = property on="Test Slider" class="Slide (strict)"("Visible"=FALSE) -> ()  [unwired: 2 in, 2 out]
              }
              frame "Exposure  **" {
                n184 = Index Array(array=w297, index=2) -> (element=w298:cluster{string[]})
                n185 = call <vilib>:"NT Read String.vi"("Name"=w300) -> ("String"=w299:string)  [unwired: 9 in, 1 out]
                n186 = Unbundle(w298) -> (w294:string[])
                n187 = Match First String(2:w294, 3:w299) -> (0:w295:i32)  [unwired: 1 out]
                n188 = property on="Test Ring" class="Ring (strict)"("Value"=w295, "Strings []"=w294) -> ()  [unwired: 2 in, 2 out]
                n189 = property on="Test Ring" class="Ring (strict)"("Visible"=TRUE) -> ()  [unwired: 2 in, 2 out]
                n190 = property on="Test Slider" class="Slide (strict)"("Visible"=FALSE) -> ()  [unwired: 2 in, 2 out]
              }
              frame "Exposure Priority  **" {
                n191 = Index Array(array=w306, index=3) -> (element=w307:cluster{string[]})
                n192 = call <vilib>:"NT Read String.vi"("Name"=w309) -> ("String"=w308:string)  [unwired: 9 in, 1 out]
                n193 = Unbundle(w307) -> (w303:string[])
                n194 = Match First String(2:w303, 3:w308) -> (0:w304:i32)  [unwired: 1 out]
                n195 = property on="Test Ring" class="Ring (strict)"("Value"=w304, "Strings []"=w303) -> ()  [unwired: 2 in, 2 out]
                n196 = property on="Test Ring" class="Ring (strict)"("Visible"=TRUE) -> ()  [unwired: 2 in, 2 out]
                n197 = property on="Test Slider" class="Slide (strict)"("Visible"=FALSE) -> ()  [unwired: 2 in, 2 out]
              }
              frame "Color Enable  **" {
                n198 = Index Array(array=w315, index=4) -> (element=w316:cluster{string[]})
                n199 = call <vilib>:"NT Read String.vi"("Name"=w318) -> ("String"=w317:string)  [unwired: 9 in, 1 out]
                n200 = Unbundle(w316) -> (w312:string[])
                n201 = Match First String(2:w312, 3:w317) -> (0:w313:i32)  [unwired: 1 out]
                n202 = property on="Test Ring" class="Ring (strict)"("Value"=w313, "Strings []"=w312) -> ()  [unwired: 2 in, 2 out]
                n203 = property on="Test Ring" class="Ring (strict)"("Visible"=TRUE) -> ()  [unwired: 2 in, 2 out]
                n204 = property on="Test Slider" class="Slide (strict)"("Visible"=FALSE) -> ()  [unwired: 2 in, 2 out]
              }
              frame Default {
                n205 = property on="Test Ring" class="Ring (strict)"("Visible"=FALSE) -> ()  [unwired: 2 in, 2 out]
                n206 = property on="Test Slider" class="Slide (strict)"("Visible"=FALSE) -> ()  [unwired: 2 in, 2 out]
              }
              frame "Brightness  **", "Color Level  **", "Compression  **", "FPS  **", "Sharpness  **" {
                n207 = call <vilib>:"NT Read Number.vi"("Name"=w324) -> ("Numeric"=w323:dbl)  [unwired: 9 in, 1 out]
                n208 = local write "Test Slider"(w323) -> ()
                n209 = property on="Test Slider" class="Slide (strict)"("Visible"=TRUE, "Scale.Maximum"=100.0 ("Scale.Range:Maximum")) -> ()  [unwired: 2 in, 2 out]
                n210 = property on="Test Ring" class="Ring (strict)"("Visible"=FALSE) -> ()  [unwired: 2 in, 2 out]
              }
            }
          }
        }
        n211 = property on="Progress" class="Clust (strict)"("Visible"=FALSE) -> ()  [unwired: 2 in, 2 out]
      }
      event "Test Name": Mouse Enter {
        # "Populate the ring with the list of tests"
        n212 = event-data() -> ()  [unwired: 1 in, 1 out]
        n213 = call <vilib>:"NT Read String Array.vi"("Name"="/TestMode/TestList") -> ("String Array"=w333:string[])  [unwired: 9 in, 1 out]
        n214 = Build Array (concatenate)("Select the test to run...", w333) -> (w332:string[])
        n215 = property on="Test Name" class="Ring (strict)"("Strings []"=w332) -> ()  [unwired: 2 in, 2 out]
      }
      event "Test Name": Value Change {
        w336 = FALSE ("Visible")
        # "Tell the robot the test name to run"
        n216 = event-data() -> ("NewVal"=w340:u16)  [unwired: 1 in]
        n217 = property on="Test Name" class="Ring (strict)"() -> ("Strings []"=w341:string[])  [unwired: 2 in, 2 out]
        n218 = local write "Progress"(T5 {"Test Progress"=0, "Test Progress Text"=""} ("Progress")) -> ()
        n219 = Index Array(array=w341, index=w340) -> (element=w339:string)
        n220 = call <vilib>:"NT Write String.vi"("String"=w339, "Name"="/TestMode/TestName") -> ()  [unwired: 9 in, 1 out]
        n221 = property on="Progress" class="Clust (strict)"("Visible"=TRUE) -> ()  [unwired: 2 in, 2 out]
        n222 = property on="Motor" class="Clust (strict)"("Visible"=w336) -> ()  [unwired: 2 in, 2 out]
        n223 = property on="Test Slider" class="Slide (strict)"("Visible"=w336) -> ()  [unwired: 2 in, 2 out]
        n224 = property on="On/Off" class="Bool (strict)"("Visible"=w336) -> ()  [unwired: 2 in, 2 out]
        n225 = property on="Rev/Fwd" class="Clust (strict)"("Visible"=w336) -> ()  [unwired: 2 in, 2 out]
        n226 = property on="Test Ring" class="Ring (strict)"("Visible"=w336) -> ()  [unwired: 2 in, 2 out]
      }
      event "Select Auto": Mouse Enter {
        # "Populate the combo box with the list of autonomous options"
        n227 = event-data() -> ()  [unwired: 1 in, 1 out]
        n228 = call <vilib>:"NT Read String Array.vi"("Name"="Auto List") -> ("String Array"=w343:string[])  [unwired: 9 in, 1 out]
        n229 = property on="Select Auto" class="CmbBox"("Strings[]"=w343) -> ()  [unwired: 2 in, 2 out]
      }
      event "Select Auto": Value Change {
        # "User modified the Auto Selection. Write to NT variable so robot knows."
        n230 = event-data() -> ("NewVal"=w347:string)  [unwired: 1 in]
        n231 = call <vilib>:"NT Write String.vi"("String"=w347, "Name"="Auto Selector") -> ()  [unwired: 9 in, 1 out]
      }
      event "Command Selection": Value Change {
        # "Get the params and show in table"
        n232 = event-data() -> ("NewVal"=w354:i32)  [unwired: 1 in]
        n233 = property on="Command Selection" class="MCListbox (strict)"() -> ("ItemNames"=w352:string[][])  [unwired: 2 in, 2 out]
        n234 = call <vilib>:"WPI_DashboardUpdate Command Params.vi"("NewVal"=w354, "Commands"=w352, "Param Tbl"=w353) -> ()  [unwired: 8 in, 1 out]
      }
      event "Execute Command": Value Change {
        # "Started one, Unique ID holds\nresponse"
        n235 = event-data() -> ()  [unwired: 1 in, 1 out]
        n236 = property on="Command Selection" class="MCListbox (strict)"() -> ("ItemNames"=w366:string[][])  [unwired: 2 in, 2 out]
        n237 = Index Array(array=w366, index (row)="Command Selection", index (col)=0) -> (element=w364:string)
        n238 = call <vilib>:"Invoke Commands.vi"("Command Params"="Command Params", "Function Name"=w364) -> ("Params"=w360:u8, "Started"=w359:bool)  [unwired: 7 in, 1 out]
        n239 = Array Subset(array="Command Params", length (row)=w360) -> (w361:string[][])  [unwired: 3 in]
        n240 = Select(t="Executing" ("Cmd Status"), s=w359, f="" ("Cmd Status")) -> (s? t:f=→"Cmd Status":string)
      }
      event "Command Selection": Double Click {
        n241 = event-data() -> ("Row"=w376:i32)  [unwired: 1 in]
        n242 = property on="Command Selection" class="MCListbox (strict)"() -> ("ItemNames"=w379:string[][])  [unwired: 2 in, 2 out]
        n243 = local read "Command Params"() -> (w374:string[][])
        n244 = Index Array(array=w379, index (row)=w376, index (col)=0) -> (element=w377:string)
        n245 = call <vilib>:"Invoke Commands.vi"("Command Params"=w374, "Function Name"=w377) -> ("Params"=w373:u8, "Started"=w368:bool)  [unwired: 7 in, 1 out]
        n246 = Array Subset(array=w374, length (row)=w373) -> (w372:string[][])  [unwired: 3 in]
        n247 = Select(t="Executing" ("Cmd Status"), s=w368, f="" ("Cmd Status")) -> (s? t:f=w369:string)
        n248 = local write "Cmd Status"(w369) -> ()
      }
      event "CheckList": Double Click {
        # "Shift clears all"
        # "Update symbols on the listbox"
        n249 = event-data() -> ("PlatMods.Shift"=w382:bool, "Row"=w384:i32)  [unwired: 1 in]
        n250 = case shown="True" w382 {
          tunnel: w384 -> [w388 _]
          tunnel: 1 -> [w387 _]
          frame False {
            n251 = property on="CheckList" class="LstBox (strict)"() -> ("Item Symbols"=w386:i32[])  [unwired: 2 in, 2 out]
            n252 = Replace Array Subset(array=w386, new element=w387, index=w388) -> (w385:i32[])
            n253 = property on="CheckList" class="LstBox (strict)"("Item Symbols"=w385) -> ()  [unwired: 2 in, 2 out]
          }
          frame True {
            w389 = 0 ("Top Row")
            n254 = property on="CheckList" class="LstBox (strict)"() -> ("Number of Rows"=w391:u32)  [unwired: 2 in, 2 out]
            n255 = Initialize Array(0, w391) -> (w390:i32[])
            n256 = property on="CheckList" class="LstBox (strict)"("Top Row"=w389, "Value"=w389, "Item Symbols"=w390) -> ()  [unwired: 2 in, 2 out]
          }
        }
      }
      event "CheckList": Key Down {
        # "Update symbols on the listbox\nLeft and right keys check and uncheck"
        n257 = event-data() -> ("VKey"=w396:T21)  [unwired: 1 in]
        n258 = case shown="\"Left\", \"Right\"" w396 {
          selector: w396 -> [w401 _]
          tunnel: eventvkey."Left" ("VKey") -> [w399 _]
          frame "Left", "Right" {
            n259 = Equal?(x=w399, y=w401) -> (x = y?=w400:bool)
            n260 = Select(t=0, s=w400, f=1) -> (s? t:f=w402:i32)
            n261 = property on="CheckList" class="LstBox (strict)"() -> ("Item Symbols"=w405:i32[])  [unwired: 2 in, 2 out]
            n262 = Replace Array Subset(array=w405, new element=w402, index="CheckList") -> (w404:i32[])
            n263 = property on="CheckList" class="LstBox (strict)"("Item Symbols"=w404) -> ()  [unwired: 2 in, 2 out]
          }
          frame Default {
          }
        }
      }
      event "DB Camera Config": Value Change {
        # "Show or hide the cluster of controls, store in ini file"
        n264 = event-data() -> ("NewVal"=w410:bool)  [unwired: 1 in]
        n265 = case shown="False" w410 {
          tunnel: w409 -> [w419 _]
          tunnel: [w412 w430] -> w408
          tunnel: w407 -> [w411 w430]
          frame False {
            w426 = "Camera"
            w429 = FALSE ("Visible")
            n266 = local read "Camera Settings"() -> (w418:T3)
            n267 = Index Array(array=w419) -> (element=w422:cluster{string[]})  [unwired: 1 in]
            n268 = Unbundle(w418) -> ("Frame Rate"=w417:i32, "Compression"=w416:i32, "Size"=w420:u16)
            n269 = Unbundle(w422) -> (w421:string[])
            n270 = Index Array(array=w421, index=w420) -> (element=w415:string)
            n271 = call-poly <vilib>:"Write Key.vi"("section"=w426, "value"=w415, "key"="Size", "refnum"=w411) -> ("refnum out"=w428:T13)  [unwired: 2 in, 5 out]
            n272 = call-poly <vilib>:"Write Key.vi"("section"=w426, "value"=w417, "key"="FrameRate", "refnum"=w428) -> ("refnum out"=w427:T13)  [unwired: 1 in, 6 out]
            n273 = property on="Camera Settings" class="Clust (strict)"("Visible"=w429) -> ()  [unwired: 2 in, 2 out]
            n274 = local write "DB Camera Config"(w429) -> ()
            n275 = call-poly <vilib>:"Write Key.vi"("section"=w426, "value"=w416, "key"="Compression", "refnum"=w427) -> ("refnum out"=w413:T13)  [unwired: 1 in, 6 out]
            n276 = call <vilib>:"Close Config Data.vi"("refnum"=w413) -> ("file path"=w414:path)  [unwired: 2 in, 8 out]
            n277 = call <vilib>:"Open Config Data.vi"("configuration file path"=w414) -> ("refnum"=w412:T13)  [unwired: 8 in, 2 out]
          }
          frame True {
            n278 = property on="Camera Settings" class="Clust (strict)"("Visible"=TRUE) -> ()  [unwired: 2 in, 2 out]
          }
        }
      }
      event "Camera Settings": Value Change {
        # "Update summary string when any elements of DB camera change"
        n279 = event-data() -> ("NewVal"=w444:T3)  [unwired: 1 in]
        n280 = Index Array(array=w440) -> (element=w439:cluster{string[]})  [unwired: 1 in]
        n281 = Unbundle(w444) -> ("Frame Rate"=w435:i32, "Compression"=w434:i32, "Size"=w437:u16)
        n282 = Unbundle(w439) -> (w438:string[])
        n283 = Index Array(array=w438, index=w437) -> (element=w436:string)
        n284 = Format Into String(format string="%s   %dfps   %d%%", w436, w435, w434) -> (resulting string=w441:string)  [unwired: 2 in, 1 out]
        n285 = Build Array(w441) -> (w442:string[])
        n286 = property on="DB Camera Config" class="Bool (strict)"("Strings [4]"=w442) -> ()  [unwired: 2 in, 2 out]
      }
      event "Motor.Enable": Value Change {
        # "When the test mode otor enable helper is set, update that\ntree row item's value"
        n287 = event-data() -> ("NewVal"=w451:bool)  [unwired: 1 in]
        n288 = Unbundle("Motor") -> ("Value"=w450:dbl)  [unwired: 1 out]
        n289 = Select(t=w450, s=w451, f=0.0) -> (s? t:f=w448:dbl)
        n290 = call <vilib>:"NT Write Number.vi"("Numeric"=w448, "Name"=w447) -> ()  [unwired: 9 in, 1 out]
      }
      event "Test Slider": Value Change {
        # "When the test mode slider helper is set, update that\ntree row item's value"
        n291 = event-data() -> ("NewVal"=w455:dbl)  [unwired: 1 in]
        n292 = call <vilib>:"NT Write Number.vi"("Numeric"=w455, "Name"=w456) -> ()  [unwired: 9 in, 1 out]
      }
      event "On/Off": Value Change {
        # "When the test mode on/off helper value is set, update that\ntree row item's value"
        n293 = event-data() -> ("NewVal"=w461:bool)  [unwired: 1 in]
        n294 = Boolean To (0,1)(Boolean=w461) -> (0, 1=w460:i16)
        n295 = call <vilib>:"NT Write Number.vi"("Numeric"=w460, "Name"=w459) -> ()  [unwired: 9 in, 1 out]
      }
      event "Rev/Fwd": Value Change {
        # "When the test mode helper value for relays is set, update that\ntree row item's value"
        n296 = event-data() -> ("NewVal.Forward"=w470:bool, "NewVal.Reverse"=w469:bool)  [unwired: 1 in]
        n297 = Boolean To (0,1)(Boolean=w470) -> (0, 1=w466:i16)
        n298 = Boolean To (0,1)(Boolean=w469) -> (0, 1=w468:i16)
        n299 = Negate(x=w468) -> (-x=w467:i16)
        n300 = Add(x=w466, y=w467) -> (x+y=w465:i16)
        n301 = call <vilib>:"NT Write Number.vi"("Numeric"=w465, "Name"=w464) -> ()  [unwired: 9 in, 1 out]
      }
      event "Test Ring": Value Change {
        # "When a test mode helper value is selected from the ring,\nset the tree item's variable to the string value"
        n302 = event-data() -> ("NewVal"=w475:u16)  [unwired: 1 in]
        n303 = property on="Test Ring" class="Ring (strict)"() -> ("Strings []"=w476:string[])  [unwired: 2 in, 2 out]
        n304 = Index Array(array=w476, index=w475) -> (element=w474:string)
        n305 = call <vilib>:"NT Write String.vi"("String"=w474, "Name"=w473) -> ()  [unwired: 9 in, 1 out]
      }
      event "Rec Mode": Value Change {
        # "Update globals for recording mode and path to read log from.\nClear when logging and let NetworkTables set path for vision to\nuse."
        n306 = event-data() -> ("NewVal"=w488:enum32{"Stop", "Record", "Playback"})  [unwired: 1 in]
        n307 = global write "WPI_DashboardLogging Global.vi" "Logging Filename"(path "") -> ()
        n308 = global write "WPI_DashboardLogging Global.vi" "Recording"(w488) -> ()
        n309 = case shown="\"Playback\"" w488 {
          tunnel: w487 -> [_ w490 w499]
          tunnel: [_ _ w498] -> w484
          tunnel: [_ _ w497] -> _
          tunnel: w482 -> [_ _ w495]
          tunnel: cluster{i32, i32} {-250, 170} -> [_ _ w494]
          tunnel: [_ _ T22 {"Image Size"=TRUE, "Image Type"=TRUE, "Pixel Value"=TRUE, "ROI Information"=TRUE, "Zoom Factor"=FALSE} ("Image Information Shown:All Elements")] -> w480
          tunnel: [_ _ TRUE ("Zoom Factor")] -> w479
          tunnel: w478 -> [_ _ w491]
          frame Default {
          }
          frame "Stop", "Record" {
            # "Place Window too"
            n310 = invoke class="VI" method="FP.Close"(reference=w490) -> (reference out=w489:refnum<vi>)  [unwired: 2 in, 2 out]
            n311 = invoke class="VI" method="Abort VI"(reference=w489) -> ()  [unwired: 2 in, 3 out]
          }
          frame "Playback" {
            n312 = call "Open Playback Panel.vi"("Offset"=w494, "DB VI Ref"=w495, "Playback in"=w499) -> ("Playback out"=w496:refnum<vi>)  [unwired: 8 in]
            n313 = register-events(w496, w491) -> (reference out=w498:refnum<event-registration>, error out=w497:errorcluster)  [unwired: 2 in]
          }
        }
        n314 = property on="Camera Image" class="ImageControl"("Image Information Shown"=w480, "Image Information Visible"=w479) -> ()  [unwired: 2 in, 2 out]
        n315 = call <vilib>:"WPI_DashboardNT Log FieldName Cache.vi"("Operation"=enum16{"Lookup/Add", "Index", "Clear"}."Clear") -> ()  [unwired: 8 in, 3 out]
      }
      event Panel Close {
        w501 = enum32{"Stop", "Record", "Playback"}."Stop" ("Rec Mode")
        # "Playback window has been closed, abort"
        n316 = event-data() -> ()  [unwired: 1 in, 4 out]
        n317 = local write "Rec Mode"(w501) -> ()
        n318 = global write "WPI_DashboardLogging Global.vi" "Recording"(w501) -> ()
      }
      event Panel Close {
        # "Abort playback window and ourself"
        n319 = event-data() -> ()  [unwired: 1 in, 4 out]
        n320 = invoke class="VI" method="FP.Close"(reference=w507) -> (reference out=w506:refnum<vi>)  [unwired: 2 in, 2 out]
        n321 = invoke class="VI" method="Abort VI"(reference=w506) -> (error out=w505:errorcluster)  [unwired: 2 in, 2 out]
        n322 = invoke class="VI" method="Abort VI"(error in=w505) -> ()  [unwired: 2 in, 3 out]
      }
      event User Event {
        n323 = event-data() -> ("IDs"=w515:cluster{"RPC field ID":u16, "Unique ID":u16}, "String"=w514:string)  [unwired: 1 in]
        n324 = Bundle("IDs"=w515, "String"=w514) -> (w513:T6)  [unwired: 1 in]
        n325 = call <vilib>:"Retrieve RPC Response.vi"("RPC Response"=w513) -> ("Output"=w510:string[][])  [unwired: 10 in]
        n326 = Build Array (concatenate)(w508, w510) -> (w509:string[][])
        n327 = local write "Command Params"(w509) -> ()
        n328 = local write "Cmd Status"("" ("Cmd Status")) -> ()
      }
      event "Vision": Value Change {
        # "Enable/Disable Compression slider.\nHW USB is hard-coded into the camera"
        n329 = event-data() -> ("NewVal"=w522:u16)  [unwired: 1 in]
        n330 = Equal?(x=w522, y=u32 2 ("milliseconds to wait")) -> (x = y?=w520:bool)
        n331 = Select(t=T23."Disabled and Grayed Out" ("Disabled"), s=w520, f=T23."Enabled" ("Disabled")) -> (s? t:f=w517:T23)
        n332 = property on="Compression" class="Slide (strict)"("DisabledEnum"=w517) -> ()  [unwired: 2 in, 2 out]
      }
      event "Tree": Double Click {
        n333 = event-data() -> ("PlatMods"=w527:T26, "Tag"=w526:string)  [unwired: 1 in]
        n334 = Unbundle(w527) -> ("Shift"=w525:bool)  [unwired: 4 out]
        n335 = Not(x=w525) -> (.not. x?=w524:bool)
        n336 = call <vilib>:"NT Update Persistence.vi"("Persistence"=w524, "Name"=w526) -> ()  [unwired: 9 in, 1 out]
      }
    }
  }
  n337 = while {
    tunnel: w47 -> [w531]
    i -> [w534]
    stop <- FALSE stop-if-true
    n338 = Wait (ms)(milliseconds to wait=u32 100) -> ()  [unwired: 1 out]
    n339 = case shown="\"Playback\"" "Rec Mode" {
      tunnel: w534 -> [_ _ w549]
      tunnel: [u32 2829099 ("Base Color") u32 11141120 ("Target Color") w538] -> w530
      frame "Stop", Default {
        # "Reset the color, extra updates don't cost much"
      }
      frame "Record" {
      }
      frame "Playback" {
        # "Playback"
        n340 = Quotient & Remainder(x=w549, y=u32 50 ("milliseconds to wait")) -> (x-y*floor(x/y)=w545:u32)  [unwired: 1 out]
        n341 = Divide(x=w545, y=u32 50 ("milliseconds to wait")) -> (x/y=w542:dbl)
        n342 = Multiply(x=6.283185307179586, y=w542) -> (x*y=w547:dbl)
        n343 = Sine(x=w547) -> (sin(x)=w546:dbl)
        n344 = Absolute Value(x=w546) -> (abs(x)=w539:dbl)
        n345 = call "Interpolate RGB Color.vi"("Proportion"=w539, "Target Color"=u32 30976, "Base Color"=u32 2829099) -> ("Result Color"=w538:u32)  [unwired: 8 in]
      }
    }
    n346 = property class="Pane"(reference=w531, "PaneColor"=w530) -> ()  [unwired: 1 in, 2 out]
  }
  n347 = local write "Dashboard Tab"(T2."Drive" ("Dashboard Tab")) -> ()
  n348 = while {
    stop <- FALSE stop-if-true
    n349 = call-poly <vilib>:"NT Write Value.vi"("Numeric"="Auto Routine", "Name"="Auto Routine") -> ()  [unwired: 9 in, 1 out]
    n350 = call-poly <vilib>:"NT Write Value.vi"("Boolean"="Shoot?", "Name"="Shoot") -> ()  [unwired: 9 in, 1 out]
    n351 = call-poly <vilib>:"NT Write Value.vi"("Numeric"="Defense", "Name"="Defense") -> ()  [unwired: 9 in, 1 out]
    n352 = call-poly <vilib>:"NT Write Value.vi"("Numeric"="Defense Position", "Name"="Defense Position") -> ()  [unwired: 9 in, 1 out]
    n353 = call-poly <vilib>:"NT Write Value.vi"("Boolean"="Cross Back", "Name"="Cross Back") -> ()  [unwired: 9 in, 1 out]
    n354 = call-poly <vilib>:"NT Write Value.vi"("Numeric"="Auto Delay (s)", "Name"="Auto Delay") -> ()  [unwired: 9 in, 1 out]
    n355 = call-poly <vilib>:"NT Write Value.vi"("Numeric"="Joystick Drive", "Name"="Joystick Drive") -> ()  [unwired: 9 in, 1 out]
    n356 = call-poly <vilib>:"NT Read Value.vi"("Name"="Gyro") -> ("Numeric"=→"Gyro":dbl)  [unwired: 9 in, 1 out]
    n357 = Wait (ms)(milliseconds to wait=u32 100) -> ()  [unwired: 1 out]
  }
  n358 = property on="On/Off" class="Bool (strict)"("Visible"=w15) -> ()  [unwired: 2 in, 2 out]
  n359 = property on="Motor" class="Clust (strict)"("Visible"=w15) -> ()  [unwired: 2 in, 2 out]
  n360 = property on="Progress" class="Clust (strict)"("Visible"=w15) -> ()  [unwired: 2 in, 2 out]
  n361 = property on="Test Ring" class="Ring (strict)"("Visible"=w15) -> ()  [unwired: 2 in, 2 out]
  n362 = property on="Rev/Fwd" class="Clust (strict)"("Visible"=w15) -> ()  [unwired: 2 in, 2 out]
  n363 = property on="Camera Settings" class="Clust (strict)"("Visible"=w15) -> ()  [unwired: 2 in, 2 out]
  n364 = local write "DB Camera Config"(w15) -> ()
  n365 = while {
    tunnel: u16 1741 ("timeout ms (25000)") -> [w569]
    stop <- FALSE stop-if-true
    n366 = TCP Create Listener(10:w569) -> (0:w568:errorcluster, 3:w570:refnum<k5>)  [unwired: 4 in, 1 out]
    n367 = case shown="No Error" w568 {
      selector: w568 -> [w572 _]
      tunnel: w570 -> [w573 _]
      frame No Error {
        n368 = while {
          tunnel: w573 -> [w576]
          tunnel: w572 -> [w575]
          stop <- FALSE stop-if-true
          n369 = TCP Wait On Listener(8:w575, 11:w576) -> (0:w577:errorcluster, 4:w578:refnum<k5>)  [unwired: 2 in, 3 out]
          n370 = local write "TCP"(w578) -> ()
          n371 = case shown="No Error" w577 {
            frame No Error {
            }
            frame Error {
              n372 = Wait (ms)(milliseconds to wait=u32 1000) -> ()  [unwired: 1 out]
            }
          }
        }
      }
      frame Error {
        n373 = Wait (ms)(milliseconds to wait=u32 1000) -> ()  [unwired: 1 out]
      }
    }
  }
  n374 = local write "Command Params"(string[][] [] ("Command Params")) -> ()
  n375 = global write "WPI_DashboardLogging Global.vi" "Recording"(w41) -> ()
  n376 = local write "Rec Mode"(w41) -> ()
  n377 = local write "Command Selection"(u16 0 ("milliseconds to wait")) -> ()
